vi "sv_Update AO Index.vi"(8 "read/write indices":T1(array[cluster]), 9 "current AO index":i32, 11 "indice computations in":T2) -> (3 "new read/write indices":T1(array[cluster]), 5 "new AO index":i32, 7 "new freq stop index":u32)   [LabVIEW 2017, in "SoundVib_SweptSine.lvlib"]
uses:
  <vilib>/addons/Sound and Vibration/svt_Swept Sine/SoundVib_SweptSine.lvlib
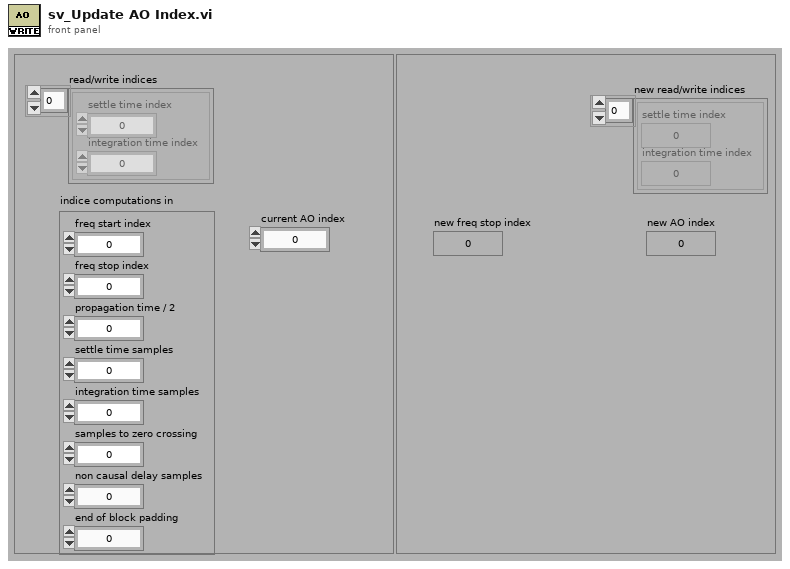
[diagram p1: front panel]
types:
  T1 = cluster{"settle time index":u32, "integration time index":u32}[]
  T2 = cluster{"freq start index":u32, "freq stop index":u32, "propagation time / 2":u32, "settle time samples":u32, "integration time samples":u32, "samples to zero crossing":u32, "non causal delay samples":u32, "end of block padding":u32}
  T3 = cluster{"settle time index":u32, "integration time index":u32}
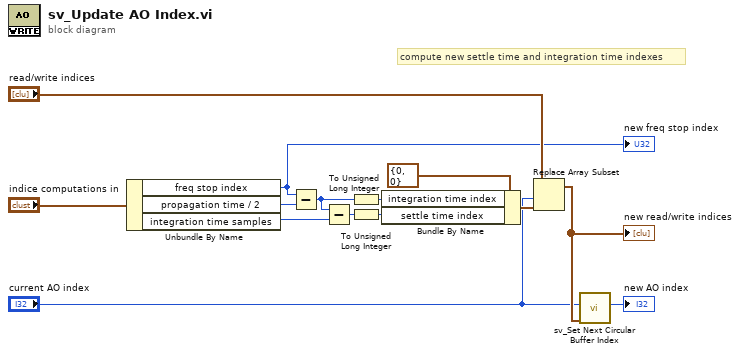
[diagram p0: block diagram]
diagram:
  # "compute new settle time and integration time indexes"
  n1 = Unbundle By Name("indice computations in") -> ("freq stop index"=w1:u32, "propagation time / 2"=w11:u32, "integration time samples"=w10:u32)
  "new freq stop index" <- w1
  n2 = Subtract(x=w1, y=w11) -> (x-y=w14:u32)
  n3 = Subtract(x=w14, y=w10) -> (x-y=w13:u32)
  n4 = To Unsigned Long Integer(number=w14) -> (unsigned 32bit integer=w4:u32)
  n5 = To Unsigned Long Integer(number=w13) -> (unsigned 32bit integer=w3:u32)
  n6 = Bundle By Name(cluster=T3 {"settle time index"=0, "integration time index"=0} ("output cluster"), "integration time index"=w4, "settle time index"=w3) -> (w8:T3)
  n7 = Replace Array Subset(array="read/write indices", new element=w8, index="current AO index") -> (w6:T1)
  "new read/write indices" <- w6
  n8 = call <vilib>:"sv_Set Next Circular Buffer Index.vi"("read/write indices"=w6, "current index"="current AO index") -> ("new index"=→"new AO index":i32)  [unwired: 9 in]
